vi "SR830 query frequency.vi"(8 "error in (no error)":errorcluster, 11 "VISA resource name":refnum<visa-resource-name>) -> (0 "error out":errorcluster, 2 "frequency":dbl[unit], 3 "VISA resource name out":refnum<visa-resource-name>)   [LabVIEW 2009, in "Lockin.lvclass"]
doc: "Reads the current frequency of the lock-in amplifier."
uses:
  Lockin.lvclass
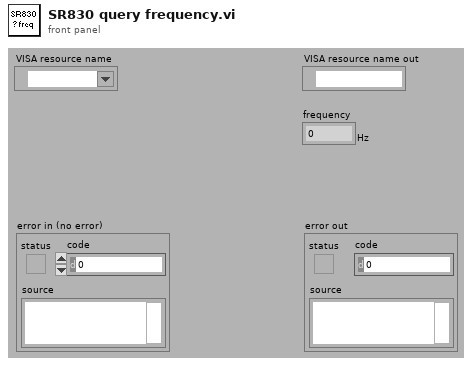
[diagram p1: front panel]
types:
  T1 = typedef "Semaphore RefNum" = refnum<k1>
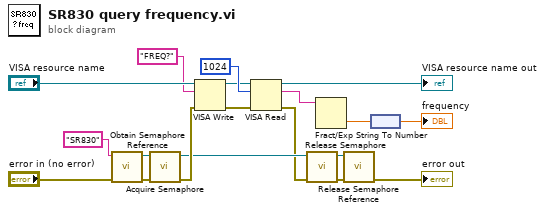
[diagram p0: block diagram]
diagram:
  n1 = call <vilib>:"Obtain Semaphore Reference.vi"("error in (no error)"="error in (no error)", "name (unnamed)"="SR830") -> ("error out"=w12:errorcluster, "semaphore"=w11:T1)  [unwired: 1 in, 3 out]
  n2 = call <vilib>:"Acquire Semaphore.vi"("error in (no error)"=w12, "semaphore"=w11) -> ("error out"=w8:errorcluster, "semaphore out"=w5:T1)  [unwired: 1 in, 3 out]
  n3 = VISA Write(VISA resource name="VISA resource name", write buffer="FREQ?", error in (no error)=w8) -> (VISA resource name out=w18:refnum<visa-resource-name>, error out=w17:errorcluster)  [unwired: 1 out]
  n4 = VISA Read(VISA resource name=w18, byte count=u32 1024 ("bytes to read (1000)"), error in (no error)=w17) -> (VISA resource name out=→"VISA resource name out":refnum<visa-resource-name>, read buffer=w13:string, error out=w4:errorcluster)  [unwired: 1 out]
  n5 = call <vilib>:"Release Semaphore.vi"("error in (no error)"=w4, "semaphore"=w5) -> ("error out"=w7:errorcluster, "semaphore out"=w6:T1)  [unwired: 4 out]
  n6 = Fract/Exp String To Number(string=w13) -> (number=w2:dbl)  [unwired: 4 out]
  n7 = call <vilib>:"Release Semaphore Reference.vi"("error in (no error)"=w7, "semaphore"=w6) -> ("error out"=→"error out":errorcluster)  [unwired: 9 out]
  n8 = node(w2) -> (→"frequency":dbl[unit])
